vi "unused_destroy.vi"(8 "error in (no error)":errorcluster, 11 "ExampleTask_StopNotifier in":refnum<class "ExampleTask_BoolUserEventStopNotifier.lvclass">) -> (0 "error out":errorcluster, 3 "loopCounter":i32)   [LabVIEW 2023]
doc: "Destructor.\nIt also returns the value of loopCounter."
uses:
  ExampleTask_BoolUserEventStopNotifier.lvclass
  ExampleTask_BoolUserEventStopNotifier.lvclass/ExampleTask_BoolUserEventStopNotifier.ctl
  unused_Read loopCounter.vi
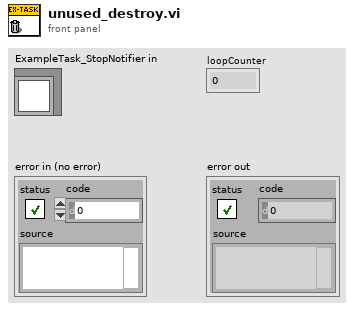
[diagram p1: front panel]
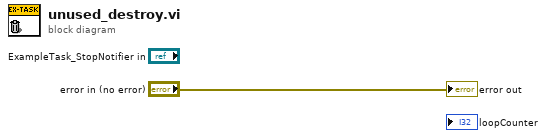
[diagram p0: block diagram]
diagram:
  "error out" <- "error in (no error)"
